vi "多反镜角度规范角数值.vi"(9 "反射镜数量":dbl=9.0 format="%#_13g", 11 "多反镜角度":dbl) -> (0 "周数":i32, 1 "规范化的角度":dbl, 3 "多反镜规范角数值":u32)   [LabVIEW 2018]
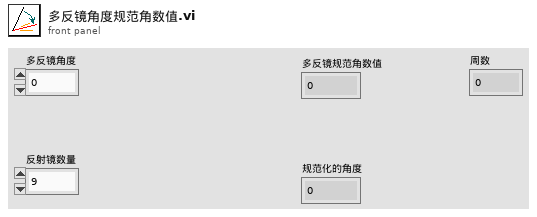
[diagram p1: front panel]
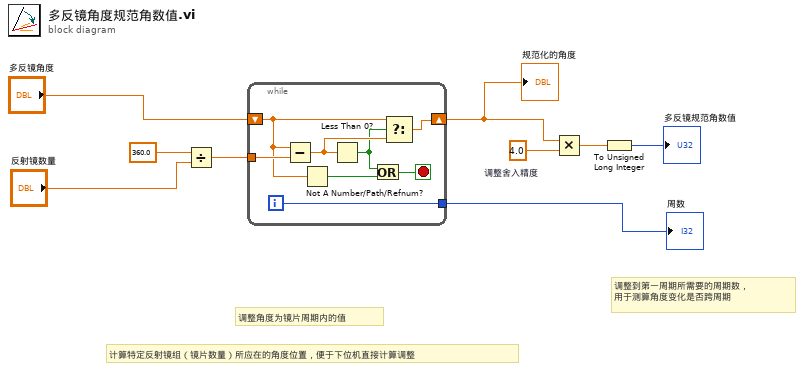
[diagram p0: block diagram]
diagram:
  w6 = 4.0  # 调整舍入精度
  # "调整到第一周期所需要的周期数，\n用于测算角度变化是否跨周期"
  # "调整角度为镜片周期内的值"
  # "计算特定反射镜组（镜片数量）所应在的角度位置，便于下位机直接计算调整"
  n1 = Divide(x=360.0, y="反射镜数量") -> (x/y=w7:dbl)
  n2 = while {
    tunnel: w7 -> [w17]
    shift-right: [w16] -> w5
    shift-left: "多反镜角度" -> [w14]
    tunnel: [w10] -> w1
    i -> [w10]
    stop <- w12 stop-if-true
    n3 = Subtract(x=w14, y=w17) -> (x-y=w15:dbl)
    n4 = Not A Number/Path/Refnum?(number/path/refnum=w14) -> (NaN/Path/Refnum?=w11:bool)
    n5 = Less Than 0?(x=w15) -> (x < 0?=w13:bool)
    n6 = Or(x=w13, y=w11) -> (x .or. y?=w12:bool)
    n7 = Select(t=w14, s=w13, f=w15) -> (s? t:f=w16:dbl)
  }
  "规范化的角度" <- w5
  "周数" <- w1
  n8 = Multiply(x=w5, y=w6) -> (x*y=w4:dbl)
  n9 = To Unsigned Long Integer(number=w4) -> (unsigned 32bit integer=→"多反镜规范角数值":u32)
